vi "Main_Host - Handle Errors.vi"(8 "error in (no error)":errorcluster) -> (3 "VI Exit?":bool)   [LabVIEW 2020]
doc: "JSMA Project Wizard 0.2.0.11\nRob Humfeld - JET Engineering\nCopyright (c) 2020, JET Engineering"
uses:
  <vilib>/Utility/error.llb/DialogType.ctl
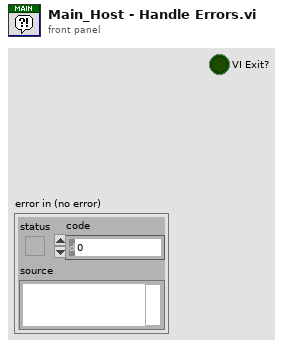
[diagram p1: front panel]
types:
  T1 = enum16{"open", "replace", "create", "open or create", "replace or create", "replace or create with confirmation"}
  T2 = typedef "DialogType.ctl" = u16
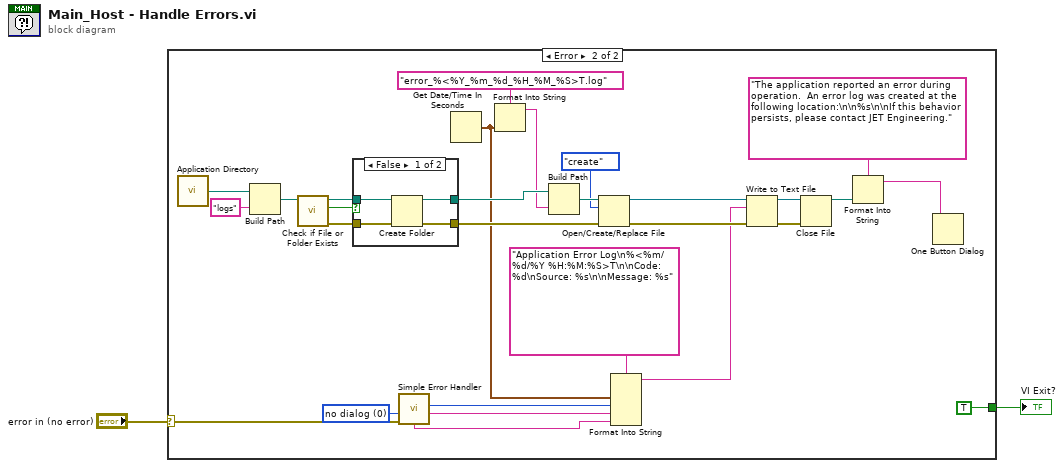
[diagram p0: block diagram]
diagram:
  n1 = case shown="Error" "error in (no error)" {
    selector: "error in (no error)" -> [_ w18]
    tunnel: [_ TRUE] -> w1
    frame No Error {
    }
    frame Error {
      w17 = T2 0 items=["no dialog", "OK message", "continue or stop message", "OK message + warnings", "continue/stop + warnings"] ("type of dialog (OK msg:1)")
      n2 = call <vilib>:"Application Directory.vi"() -> ("Application Directory"=w30:path)
      n3 = Build Path(base path=w30, name or relative path="logs") -> (appended path=w28:path)
      n4 = call <vilib>:"Check if File or Folder Exists.vi"("path"=w28) -> ("error out"=w25:errorcluster, "file or folder exists?"=w27:bool, "dup path"=w26:path)  [unwired: 8 in]
      n5 = case shown="False" w27 {
        tunnel: w26 -> [w33 w36]
        tunnel: [w32 w36] -> w22
        tunnel: w25 -> [w34 w35]
        tunnel: [w31 w35] -> w24
        frame False {
          n6 = Create Folder(path (use dialog)=w33, error in=w34) -> (created path=w32:path, error out=w31:errorcluster)  [unwired: 1 in, 1 out]
        }
        frame True {
        }
      }
      n7 = call <vilib>:"Simple Error Handler.vi"("type of dialog (OK msg:1)"=w17, "error in (no error)"=w18) -> ("code out"=w14:i32, "source out"=w13:string, "message"=w12:string)  [unwired: 3 in, 2 out]
      n8 = Get Date/Time In Seconds() -> (seconds since 1Jan1904=w15:timestamp)
      n9 = Format Into String(format string="error_%<%Y_%m_%d_%H_%M_%S>T.log", w15) -> (resulting string=w21:string)  [unwired: 2 in, 1 out]
      n10 = Build Path(base path=w22, name or relative path=w21) -> (appended path=w20:path)
      n11 = Open/Create/Replace File(file path (use dialog)=w20, error in=w24, operation (0:open)=T1."create") -> (refnum out=w10:refnum<file>, error out=w11:errorcluster)  [unwired: 3 in, 1 out]
      n12 = Format Into String(format string="Application Error Log\n%<%m/%d/%Y %H:%M:%S>T\n\nCode: %d\nSource: %s\n\nMessage: %s", w15, w14, w13, w12) -> (resulting string=w9:string)  [unwired: 2 in, 1 out]
      n13 = Write to Text File(file (use dialog)=w10, text=w9, error in=w11) -> (refnum out=w7:refnum<file>, error out=w8:errorcluster)  [unwired: 1 in, 1 out]
      n14 = Close File(refnum=w7, error in=w8) -> (path=w6:path)  [unwired: 1 out]
      n15 = Format Into String(format string="The application reported an error during operation.  An error log was created at the following location:\n\n%s\n\nIf this behavior persists, please contact JET Engineering.", w6) -> (resulting string=w3:string)  [unwired: 2 in, 1 out]
      n16 = One Button Dialog(message=w3) -> ()  [unwired: 1 in, 1 out]
    }
  }
  "VI Exit?" <- w1
